vi "Close SHVs.vi"(8 "error in (no error)":errorcluster, 11 "cRIO-CO2 in":refnum<class "cRIO-CO2.lvclass">) -> (0 "error out":errorcluster, 3 "cRIO-CO2 out":refnum<class "cRIO-CO2.lvclass">)   [LabVIEW 2015, in "cRIO-Carbondioxide.lvlib" / "cRIO-CO2.lvlib" / "cRIO-CO2.lvclass"]
uses:
  cRIO-CO2.lvclass
  cRIO-CO2.lvclass/cRIO-CO2.ctl
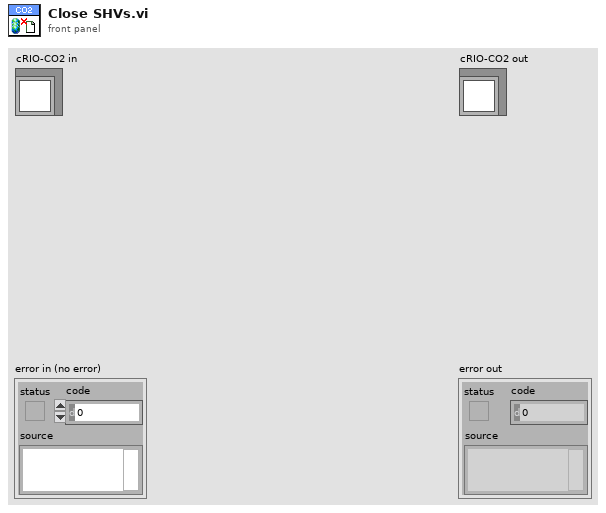
[diagram p1: front panel]
types:
  T1 = cluster{"State":refnum<k21>, "Source":refnum<k21>, "Target":refnum<k21>, "Control":refnum<k21>, "Progress":refnum<k21>}
  T2 = cluster{"State":refnum<k21>, "Push Time":refnum<k21>, "Control":refnum<k21>, "Progress":refnum<k21>}
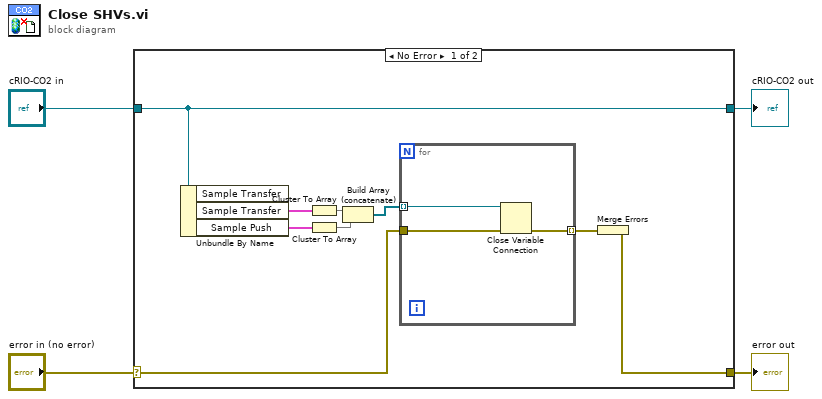
[diagram p0: block diagram]
diagram:
  n1 = case shown="No Error" "error in (no error)" {
    selector: "error in (no error)" -> [w8 w18]
    tunnel: [w11 w18] -> w3
    tunnel: [w13 w17] -> w1
    tunnel: "cRIO-CO2 in" -> [w13 w17]
    frame No Error {
      n2 = Unbundle By Name(w13) -> ("Sample Transfer"=w7:T1, "Sample Push"=w6:T2)  [unwired: 1 out]
      n3 = Cluster To Array(cluster=w7) -> (array=w9:refnum<k21>[])
      n4 = Cluster To Array(cluster=w6) -> (array=w5:refnum<k21>[])
      n5 = Build Array (concatenate)(w9, w5) -> (w10:refnum<k21>[])
      n6 = for {
        tunnel: w10 -> [w14] mode=indexing
        tunnel: w8 -> [w15]
        tunnel: [w16] -> w12 mode=indexing
        n7 = Close Variable Connection(8:w15, 11:w14) -> (0:w16:errorcluster)
      }
      n8 = Merge Errors(w12) -> (w11:errorcluster)
    }
    frame Error {
    }
  }
  "error out" <- w3
  "cRIO-CO2 out" <- w1
